vi "poly_lock_fp_updates_lock_caller.vi"(8 "error in":errorcluster) -> (0 "error out":errorcluster)   [LabVIEW 2015]
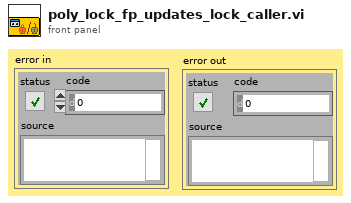
[diagram p1: front panel]
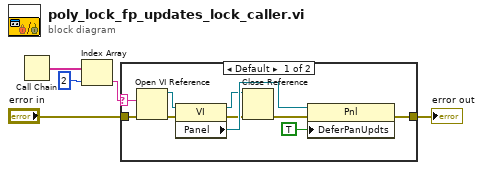
[diagram p0: block diagram]
diagram:
  n1 = Call Chain() -> (call chain=w3:string[])
  n2 = Index Array(array=w3, index=2) -> (element=w1:string)
  n3 = case shown="Default" w1 {
    selector: w1 -> [w12 _]
    tunnel: [w14 w16] -> w5
    tunnel: "error in" -> [w10 w16]
    frame Default {
      n4 = Open VI Reference(vi path=w12, error in (no error)=w10) -> (vi reference=w11:refnum<vi>, error out=w9:errorcluster)  [unwired: 4 in]
      n5 = property class="VI"(reference=w11, error in=w9) -> (reference out=w8:refnum<vi>, error out=w7:errorcluster, "Panel"=w13:refnum<vi>)
      n6 = Close Reference(reference=w8, error in (no error)=w7) -> (error out=w6:errorcluster)
      n7 = property class="Pnl"(reference=w13, error in=w6, "DeferPanUpdts"=TRUE) -> (error out=w14:errorcluster)  [unwired: 1 out]
    }
    frame "" {
      # "Skip if caller has no caller"
    }
  }
  "error out" <- w5
